vi "Close MeasurementLink Session.vi"(8 "error in":errorcluster, 9 "initialize and close session behavior":T1, 10 "session in":variant, 11 "session factory in":refnum<class "Session Factory.lvclass">) -> (0 "error out":errorcluster)   [LabVIEW 2020, in "niDMM Sessions.lvlib" / "Session Factory.lvclass"]
uses:
  Session Factory.lvclass
  Instrument Sessions/ISession Factory/Initialize and Close Session Behavior.ctl
  Instrument Sessions/ISession Factory/ISession Factory.lvclass
  <instrlib>/niDMM/nidmm.llb/niDMM Close.vi
  <instrlib>/niDMM/nidmm.llb/niDMM Detach gRPC Session.vi
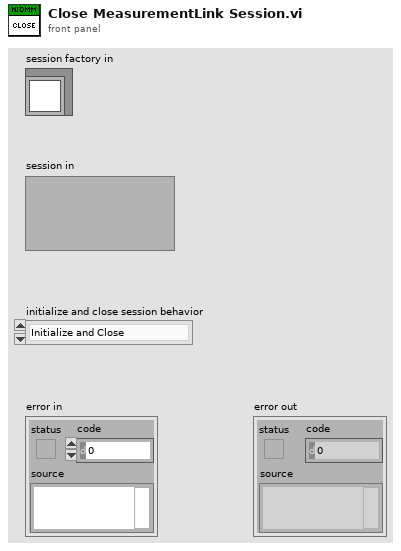
[diagram p1: front panel]
types:
  T1 = typedef "Plug-In SDK Instrument Sessions.lvlib/ISession Factory.lvclass/Initialize and Close Session Behavior.ctl" = enum16{"Initialize and Close", "Attach and Detach", "Initialize and Detach", "Attach and Close"}
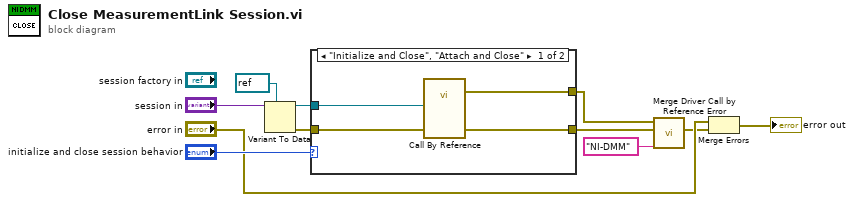
[diagram p0: block diagram]
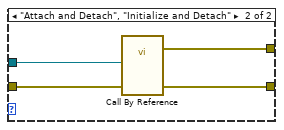
[diagram p2: hidden frame]
diagram:
  n1 = Variant To Data(type=refnum<k15> refnum ("instrument handle"), Variant="session in") -> (data=w8:refnum<k15>, error out=w9:errorcluster)  [unwired: 1 in]
  n2 = case shown="\"Initialize and Close\", \"Attach and Close\"" "initialize and close session behavior" {
    tunnel: w9 -> [w15 w19]
    tunnel: w8 -> [w14 w17]
    tunnel: [w13 w18] -> w3
    tunnel: [w12 w16] -> w2
    frame "Initialize and Close", "Attach and Close" {
      n3 = call-by-ref "?"("error in (no error)"=w15, "instrument handle"=w14) -> (error out=w12:errorcluster, 0:"error out"=w13:errorcluster)  [unwired: 11 in, 1 out]
    }
    frame "Attach and Detach", "Initialize and Detach" {
      n4 = call-by-ref "?"("error in (no error)"=w19, "instrument handle"=w17) -> (error out=w16:errorcluster, 0:"error out"=w18:errorcluster)  [unwired: 11 in, 1 out]
    }
  }
  n5 = call "Merge Driver Call by Reference Error.vi"("driver name"="NI-DMM", "called vi error"=w3, "call by ref error"=w2) -> ("error out"=w1:errorcluster)  [unwired: 8 in]
  n6 = Merge Errors("error in", w1) -> (→"error out":errorcluster)
